vi "GetISI.vi"(8 "Criterion for Burst":dbl, 10 "Raster plot":cluster{"location":dbl[], "Sweep":i32[]}[](array[cluster]), 11 "Number of Spike (1D)":i32[](array[numeric])) -> (0 "Result Table":dbl[][](array[numeric]), 2 "Pooled ISI":dbl[](array[numeric]), 3 "Train duration (1D)":string[](array[string]))   [LabVIEW 2017]
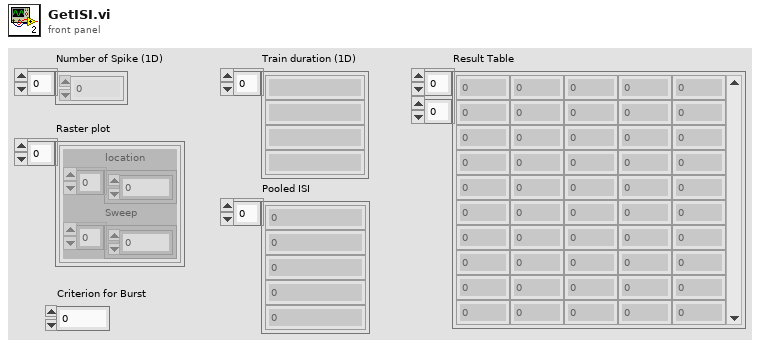
[diagram p1: front panel]
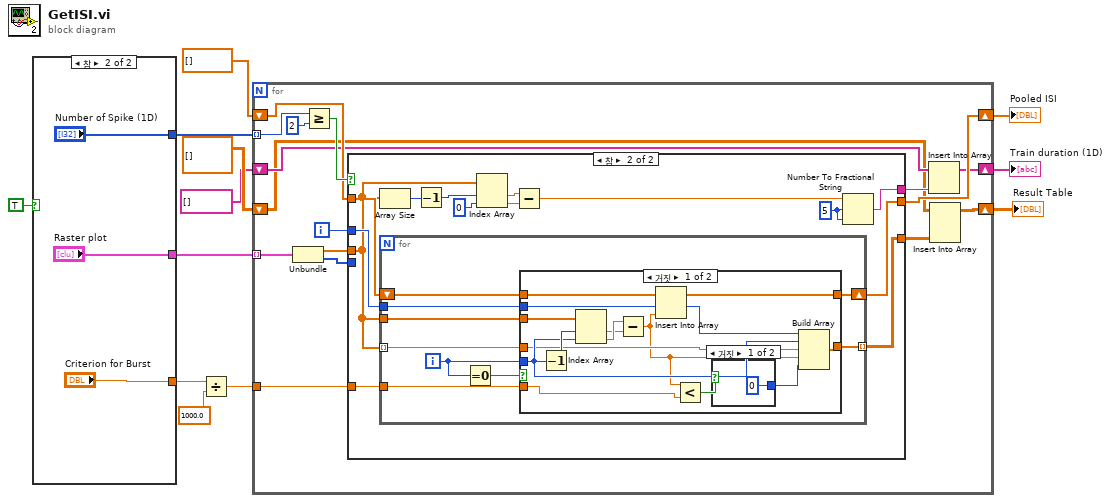
[diagram p0: block diagram]
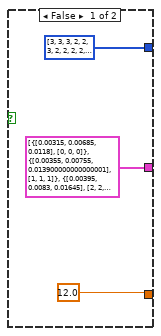
[diagram p2: hidden frame]
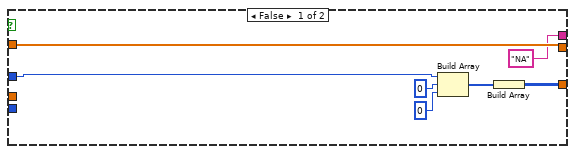
[diagram p3: hidden frame]
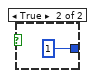
[diagram p4: hidden frame]
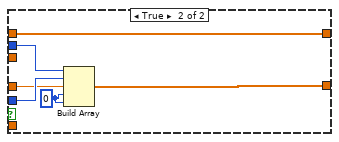
[diagram p5: hidden frame]
diagram:
  n1 = case shown="참" TRUE {
    tunnel: [i32[] [3, 3, 3, 2, 2, 3, 2, 2, 2, 2, 2, 2] ("배열 2") "Number of Spike (1D)"] -> w12
    tunnel: [cluster{"location":dbl[], "Sweep":i32[]}[] [{"location"=[0.00315, 0.00685, 0.0118], "Sweep"=[0, 0, 0]}, {"location"=[0.00355, 0.00755, 0.013900000000000001], "Sweep"=[1, 1, 1]}, {"location"=[0.00395, 0.0083, 0.01645], "Sweep"=[2, 2, 2]}, {"location"=[0.0041, 0.00885], "Sweep"=[3, 3]}, {"location"=[0.0043, 0.00885], "Sweep"=[4, 4]}, {"location"=[0.0045000000000000005, 0.009000000000000001, 0.02025], "Sweep"=[5, 5, 5]}, {"location"=[0.0046500000000000005, 0.0099], "Sweep"=[6, 6]}, {"location"=[0.00485, 0.00975], "Sweep"=[7, 7]}, {"location"=[0.005050000000000001, 0.01025], "Sweep"=[8, 8]}, {"location"=[0.00515, 0.00995], "Sweep"=[9, 9]}, {"location"=[0.00525, 0.010450000000000001], "Sweep"=[10, 10]}, {"location"=[0.0054, 0.010400000000000001], "Sweep"=[11, 11]}] ("배열 2") "Raster plot"] -> w11
    tunnel: [12.0 "Criterion for Burst"] -> w3
    frame False {
    }
    frame True {
    }
  }
  n2 = Divide(x=w3, y=1000.0) -> (x/y=w1:dbl)
  n3 = for {
    tunnel: w11 -> [w34] mode=indexing
    shift-right: [w29] -> w7
    shift-left: dbl[] [] -> [w28]
    tunnel: w12 -> [w32] mode=indexing
    shift-right: [w26] -> w6
    shift-left: string[] [] -> [w25]
    shift-right: [w22] -> w4
    shift-left: dbl[][] [] -> [w21]
    tunnel: w1 -> [w19]
    i -> [w24]
    n4 = Unbundle(w34) -> ("location"=w33:dbl[], "Sweep"=w20:i32[])
    n5 = Greater Or Equal?(x=w32, y=2) -> (x >= y?=w30:bool)
    n6 = case shown="참" w30 {
      tunnel: w33 -> [_ w43]
      tunnel: w28 -> [w41 w45]
      tunnel: [w41 w44] -> w29
      tunnel: ["NA" w50] -> w27
      tunnel: w24 -> [w39 w48]
      tunnel: [w35 w47] -> w23
      tunnel: w20 -> [_ _]
      tunnel: w19 -> [_ w42]
      frame False {
        n7 = Build Array(w39, 0 ("원소"), 0 ("원소")) -> (w36:i32[])
        n8 = Build Array(w36) -> (w35:i32[][])
      }
      frame True {
        w49 = i16 5 ("폭(-)")
        n9 = Array Size(array=w43) -> (size(s)=w46:i32)
        n10 = for {
          tunnel: w43 -> [w64]
          tunnel: w48 -> [w63]
          tunnel: [w62] -> w47 mode=indexing
          shift-right: [w58] -> w44
          shift-left: w45 -> [w59]
          tunnel: w43 -> [w57] mode=indexing
          tunnel: w42 -> [w56]
          i -> [w61]
          n11 = Equal To 0?(x=w61) -> (x = 0?=w60:bool)
          n12 = case shown="거짓" w60 {
            tunnel: w64 -> [w78 _]
            tunnel: w63 -> [w75 w86]
            tunnel: [w74 w84] -> w62
            tunnel: w61 -> [w72 w85]
            tunnel: w59 -> [w71 w83]
            tunnel: [w70 w83] -> w58
            tunnel: w57 -> [w69 w82]
            tunnel: w56 -> [w67 _]
            frame False {
              n13 = Decrement(x=w72) -> (x-1=w73:i32)
              n14 = Index Array(array=w78, index #1=w73, index #2=w72) -> (element #1=w76:dbl, element #2=w77:dbl)
              n15 = Subtract(x=w77, y=w76) -> (x-y=w68:dbl)
              n16 = Insert Into Array(array=w71, new element=w68) -> (w70:dbl[])  [unwired: 1 in]
              n17 = Less?(x=w68, y=w67) -> (x < y?=w66:bool)
              n18 = case shown="거짓" w66 {
                tunnel: [0 1] -> w65
                frame False {
                }
                frame True {
                }
              }
              n19 = Build Array(w75, w72, w69, w68, w65) -> (w74:dbl[])
            }
            frame True {
              w81 = 0 ("원소")
              n20 = Build Array(w86, w85, w82, w81, w81) -> (w84:dbl[])
            }
          }
        }
        n21 = Decrement(x=w46) -> (x-1=w55:i32)
        n22 = Index Array(array=w43, index #1=w55, index #2=0 ("인덱스")) -> (element #1=w53:dbl, element #2=w52:dbl)
        n23 = Subtract(x=w53, y=w52) -> (x-y=w51:dbl)
        n24 = Number To Fractional String(number=w51, width (-)=w49, precision (6)=w49) -> (F-format string=w50:string)  [unwired: 1 in]
      }
    }
    n25 = Insert Into Array(array=w25, new element=w27) -> (w26:string[])  [unwired: 1 in]
    n26 = Insert Into Array(array=w21, new element=w23) -> (w22:dbl[][])  [unwired: 2 in]
  }
  "Pooled ISI" <- w7
  "Train duration (1D)" <- w6
  "Result Table" <- w4
